vi "Main Tclk.vi"() -> ()   [LabVIEW 2018] (continued)
                          tunnel: w6883 -> [w6889 w6893]
                          tunnel: w6882 -> [w6888 w6892]
                          tunnel: [w6886 w6891] -> w6881
                          tunnel: [w6887 w6890] -> w6880
                          tunnel: w6867 -> [w6885 _]
                          tunnel: w6863 -> [w6884 _]
                          frame False {
                            n2158 = Build Array (concatenate)(w6885, w6889) -> (w6886:sgl[])
                            n2159 = Build Array (concatenate)(w6884, w6888) -> (w6887:sgl[][][])
                            n2160 = local write "FI grid array"(w6887) -> ()
                            n2161 = local write "FI array"(w6886) -> ()
                          }
                          frame True {
                            n2162 = Build Array(w6893) -> (w6891:sgl[])
                            n2163 = Build Array(w6892) -> (w6890:sgl[][][])
                            n2164 = local write "FI array"(w6891) -> ()
                            n2165 = local write "FI grid array"(w6890) -> ()
                          }
                        }
                      }
                    }
                  }
                }
                n2166 = local write "FI array tiled"(w6834) -> ()
                n2167 = local write "FI grid array tiled"(w6833) -> ()
              }
              frame #23 {
                w6915 = 1000 ("sample length")
                n2168 = local read "SEM Options"() -> (w6920:T27)
                n2169 = Unbundle By Name(w6920) -> ("Upload"=w6919:bool)
                n2170 = local read "Smart upload fail"() -> (w6943:bool)
                n2171 = local read "Milling Z voltage array"() -> (w6914:sgl[])
                n2172 = local read "Milling Z voltage (V)"() -> (w6922:sgl)
                n2173 = Compound Arithmetic op=AND(w6919, "Smart upload", w6943) -> (w6944:bool)
                n2174 = Build Array (concatenate)(w6914, w6922) -> (w6941:sgl[])
                n2175 = case shown="True" w6944 {
                  frame False {
                  }
                  frame True {
                    n2176 = local read "SEM Scan Parameters"() -> (w6949:T26)
                    n2177 = shared-variable ".\\Zeiss Library.lvlib\\Timestamp"() -> (w6950:timestamp)  [unwired: 1 in, 1 out]
                    n2178 = Unbundle By Name(w6949) -> ("Frames"=w6946:u8, "Y tiles"=w6948:u8, "X tiles"=w6947:u8)
                    n2179 = for {
                      N: w6946 -> [_]
                      tunnel: w6950 -> [w6954]
                      tunnel: w6948 -> [w6953]
                      tunnel: w6947 -> [w6952]
                      i -> [w6951]
                      n2180 = for {
                        N: w6953 -> [_]
                        tunnel: w6952 -> [w6958]
                        tunnel: w6954 -> [w6956]
                        tunnel: w6951 -> [w6955]
                        i -> [w6957]
                        n2181 = for {
                          N: w6958 -> [_]
                          tunnel: w6957 -> [w6965]
                          tunnel: w6956 -> [w6962]
                          tunnel: w6955 -> [w6961]
                          i -> [w6964]
                          w6960 = "-" ("string")
                          w6987 = "^" ("replace string (\"\")")
                          w6967 = "_" ("string")
                          n2182 = local read "Hardware Configuration"() -> (w6997:T25)
                          n2183 = local read "File Information"() -> (w6999:T31)
                          n2184 = Format Into String(w6961) -> (resulting string=w6959:string)  [unwired: 3 in, 1 out]
                          n2185 = Format Into String(w6965) -> (resulting string=w6966:string)  [unwired: 3 in, 1 out]
                          n2186 = Format Into String(w6964) -> (resulting string=w6963:string)  [unwired: 3 in, 1 out]
                          n2187 = Unbundle By Name(w6997) -> ("Machine ID"=w6996:string)
                          n2188 = Format Date/Time String(time format string (%c)="%y-%m-%d_%H%M%S", seconds (now)=w6962) -> (date/time string=w7002:string)  [unwired: 1 out]
                          n2189 = local read "SEM Options"() -> (w6982:T27)
                          n2190 = Unbundle By Name(w6999) -> ("Sample ID"=w6984:string, "File path"=w6998:path)
                          n2191 = Format Date/Time String(time format string (%c)="Y%Y\\M%m\\D%d", seconds (now)=w6962) -> (date/time string=w7007:string)  [unwired: 1 out]
                          n2192 = xnode "Match Regular Expression"("input string"=w6996, "regular expression"="/") -> ("after match"=w7006:string)  [unwired: 4 in, 4 out]
                          n2193 = Concatenate Strings(w7006, w6967, w7002, w6967, w6959, w6960, w6966, w6960, w6963, ".dat" ("string")) -> (w7008:string)
                          n2194 = Unbundle By Name(w6982) -> ("Delete after upload"=w6981:bool)
                          n2195 = Build Path(base path=w6998, name or relative path=w7007) -> (appended path=w7004:path)
                          n2196 = Build Path(base path=w7004, name or relative path=w7008) -> (appended path=w6983:path)
                          n2197 = Path To String(path=w6983) -> (string=w6990:string)
                          n2198 = shared-variable ".\\Zeiss Library.lvlib\\Upload flags path"() -> (w6969:string)  [unwired: 1 in, 1 out]
                          n2199 = Search and Replace String(replace all?=TRUE ("replace all? (F)"), input string=w6990, search string="\\", replace string=w6987) -> (result string=w6986:string)  [unwired: 4 in, 3 out]
                          n2200 = Select(t="^delete" ("replace string (\"\")"), s=w6981, f="^keep" ("replace string (\"\")")) -> (s? t:f=w6995:string)
                          n2201 = Search and Replace String(input string=w6986, search string=":", replace string=w6987) -> (result string=w6991:string)  [unwired: 5 in, 3 out]
                          n2202 = String To Path(string=w6969) -> (path=w6968:path)
                          n2203 = Concatenate Strings(w6984, "^" ("string"), w6991, w6995) -> (w6970:string)
                          n2204 = Build Path(base path=w6968, name or relative path="Filtered") -> (appended path=w6975:path)
                          n2205 = Build Path(base path=w6968, name or relative path=w6970) -> (appended path=w6980:path)
                          n2206 = File/Directory Info(path=w6975) -> (path out=w6973:path, error out=w6974:errorcluster)  [unwired: 1 in, 5 out]
                          n2207 = File/Directory Info(path=w6980) -> (path out=w6979:path, error out=w6978:errorcluster)  [unwired: 1 in, 5 out]
                          n2208 = Unbundle By Name(w6974) -> ("status"=w6972:bool)
                          n2209 = Unbundle By Name(w6978) -> ("status"=w6977:bool)
                          n2210 = case shown="True" w6972 {
                            tunnel: w6973 -> [w7009 w7011]
                            tunnel: [w7009 w7010] -> w6971
                            frame False {
                            }
                            frame True {
                              n2211 = Create Folder(path (use dialog)=w7011) -> (created path=w7010:path)  [unwired: 2 in, 2 out]
                            }
                          }
                          n2212 = case shown="False" w6977 {
                            tunnel: w6979 -> [w7015 _]
                            tunnel: w6971 -> [w7013 _]
                            tunnel: w6970 -> [w7012 _]
                            frame False {
                              n2213 = Build Path(base path=w7013, name or relative path=w7012) -> (appended path=w7014:path)
                              n2214 = Move(source path=w7015, 10:w7014) -> ()  [unwired: 3 in, 3 out]
                            }
                            frame True {
                            }
                          }
                        }
                      }
                    }
                  }
                }
                n2215 = local write "Milling Z voltage array"(w6941) -> ()
                n2216 = Array Size(array=w6941) -> (size(s)=w6916:i32)
                n2217 = Subtract(x=w6916, y=w6915) -> (x-y=w6940:i32)
                n2218 = Max & Min(x=w6916, y=w6915) -> (min(x,y)=w6917:i32)  [unwired: 1 out]
                n2219 = Array Subset(array=w6941, index=w6940, length=w6917) -> (w6942:sgl[])
                n2220 = for {
                  N: w6917 -> [_]
                  tunnel: [w6945] -> w6918 mode=indexing
                  i -> [w6945]
                }
                n2221 = call <vilib>:"Linear Fit.vi"("Y"=w6942, "X"=w6918) -> ("slope"=w6937:dbl)  [unwired: 9 in, 4 out]
                n2222 = local read "Milling para"() -> (w6935:T35)
                n2223 = local read "FIB Scan Parameters"() -> (w6938:T32)
                n2224 = Greater Or Equal?(x=w6916, y=100.0) -> (x >= y?=w6929:bool)
                n2225 = Unbundle By Name(w6935) -> ("FIB FOV (um)"=w6934:sgl)
                n2226 = Unbundle By Name(w6938) -> ("Z size (V)"=w6936:dbl)
                n2227 = Select(t=T44."Enabled" ("Disabled"), s=w6929, f=T44."Disabled and Grayed Out" ("Disabled")) -> (s? t:f=w6928:T44)
                n2228 = Divide(x=w6937, y=w6936) -> (x/y=w6933:dbl)
                n2229 = Compound Arithmetic op=MULTIPLY(w6934, sgl -1000.0 ("value"), w6933) -> (w6923:dbl)
                "Delta Z (nm)" <- w6923
                n2230 = property on="Delta Z (nm)" class="DigNum (strict)"("DisabledEnum"=w6928) -> ()  [unwired: 2 in, 2 out]
                n2231 = local read "Delta Z array"() -> (w6925:sgl[])
                n2232 = local read "SEM Specimen I array"() -> (w6927:sgl[])
                n2233 = local read "SEM Specimen I"() -> (w6894:dbl)
                n2234 = Build Array (concatenate)(w6925, w6923) -> (w6924:dbl[])
                n2235 = local write "Delta Z array"(w6924) -> ()
                n2236 = Build Array (concatenate)(w6927, w6894) -> (w6926:dbl[])
                n2237 = local write "SEM Specimen I array"(w6926) -> ()
                n2238 = local read "3D FIB-SEM Files"() -> (w6898:path)
                n2239 = local read "SEM Scan Parameters"() -> (w6903:T26)
                n2240 = Unbundle By Name(w6903) -> ("Y tiles"=w6906:u8, "X tiles"=w6904:u8)
                n2241 = Build Array(w6906, w6904) -> (w6905:u8[])
                n2242 = Quotient & Remainder(x=w6905, y=2) -> (floor(x/y)=w6901:i32[])  [unwired: 1 out]
                n2243 = Index Array(array=w6901) -> (element #1=w6912:i32, element #2=w6913:i32)  [unwired: 2 in]
                n2244 = Format Into String(w6912) -> (resulting string=w6911:string)  [unwired: 3 in, 1 out]
                n2245 = Format Into String(w6913) -> (resulting string=w6909:string)  [unwired: 3 in, 1 out]
                n2246 = Concatenate Strings("Low res_" ("string"), w6911, "-" ("string"), w6909, ".png" ("string")) -> (w6900:string)
                n2247 = Build Path(base path=w6898, name or relative path=w6900) -> (appended path=w6897:path)
                n2248 = Build Path(base path=w6898, name or relative path="Low res.png" ("string")) -> (appended path=w6896:path)
                n2249 = Copy(9:TRUE ("overwrite (F)"), 10:w6896, 11:w6897) -> ()  [unwired: 2 in, 3 out]
              }
              frame #24 {
                n2250 = local read "SEM Scan Parameters"() -> (w7139:T26)
                n2251 = local read "Auto re-engage"() -> (w7140:bool)
                n2252 = local read "Reheat from last"() -> (w7136:bool)
                n2253 = Unbundle By Name(w7139) -> ("Pixel size (nm)"=w7138:sgl, "Y tiles"=w7132:u8, "X tiles"=w7131:u8)
                n2254 = expression code="x/1000"(w7138) -> (w7137:sgl)
                n2255 = Build Array(w7132, w7131) -> (w7134:u8[])
                n2256 = Quotient & Remainder(x=w7134, y=2) -> (floor(x/y)=w7127:i32[])  [unwired: 1 out]
                n2257 = Index Array(array=w7127) -> (element #1=w7130:i32, element #2=w7129:i32)  [unwired: 2 in]
                n2258 = local read "Low res scale tiled"() -> (w7135:dbl[][])
                n2259 = Index Array(array=w7135, index (row)=w7130, index (col)=w7129) -> (element=w7128:dbl)
                n2260 = case shown="False" w7140 {
                  tunnel: w7137 -> [_ w7185]
                  tunnel: w7128 -> [_ w7184]
                  frame False {
                    n2261 = local read "Re-engage counts"() -> (w7160:u8)
                    n2262 = local read "Last re-engage count"() -> (w7162:u8)
                    n2263 = Less?(x=w7160, y=w7162) -> (x < y?=w7161:bool)
                    n2264 = case shown="True" w7161 {
                      tunnel: w7160 -> [_ w7171]
                      tunnel: w7160 -> [_ w7172]
                      frame False {
                      }
                      frame True {
                        n2265 = local read "Delta X"() -> (w7164:dbl)
                        n2266 = local read "Re-engage X shift array"() -> (w7173:dbl[])
                        n2267 = local read "SEM Scan Parameters"() -> (w7178:T26)
                        n2268 = local read "Delta Y"() -> (w7167:dbl)
                        n2269 = local read "Re-engage Y shift array"() -> (w7174:dbl[])
                        n2270 = Decrement(x=w7172) -> (x-1=w7166:u8)
                        n2271 = Decrement(x=w7171) -> (x-1=w7169:u8)
                        n2272 = Unbundle By Name(w7178) -> ("Pixel size (nm)"=w7179:sgl)
                        n2273 = Index Array(array=w7173, index=w7166) -> (element=w7165:dbl)
                        n2274 = Index Array(array=w7174, index=w7169) -> (element=w7170:dbl)
                        n2275 = expression code="x/1000"(w7179) -> (w7176:sgl)
                        n2276 = Divide(x=w7165, y=w7176) -> (x/y=w7163:dbl)
                        n2277 = Divide(x=w7170, y=w7176) -> (x/y=w7168:dbl)
                        n2278 = Subtract(x=w7164, y=w7163) -> (x-y=w7177:dbl)
                        n2279 = Subtract(x=w7167, y=w7168) -> (x-y=w7175:dbl)
                        n2280 = local read "Re-engage Delta X array"() -> (w7183:dbl[])
                        n2281 = local read "Re-engage Delta Y array"() -> (w7180:dbl[])
                        n2282 = Build Array (concatenate)(w7183, w7177) -> (w7182:dbl[])
                        n2283 = Build Array (concatenate)(w7180, w7175) -> (w7181:dbl[])
                        n2284 = local write "Re-engage Delta X array"(w7182) -> ()
                        n2285 = local write "Re-engage Delta Y array"(w7181) -> ()
                      }
                    }
                  }
                  frame True {
                    n2286 = local read "Re-engage Files"() -> (w7186:path)
                    n2287 = stacked-sequence {
                      tunnel: w7186 -> [w7187 w7214]
                      tunnel: w7185 -> [_ w7199]
                      tunnel: w7184 -> [_ w7198]
                      frame #0 {
                        n2288 = Build Path(base path=w7187, name or relative path="post.png " ("command line")) -> (appended path=w7192:path)
                        n2289 = local read "3D FIB-SEM Files"() -> (w7190:path)
                        n2290 = Build Path(base path=w7190, name or relative path="Low res.png " ("command line")) -> (appended path=w7191:path)
                        n2291 = Copy(9:TRUE ("run minimized? (F)"), 10:w7192, 11:w7191) -> ()  [unwired: 2 in, 3 out]
                      }
                      frame #1 {
                        n2292 = local read "SEM Options"() -> (w7220:T27)
                        n2293 = Unbundle By Name(w7220) -> ("Inverse PNG"=w7219:bool)
                        n2294 = call "SIFT align.vi"("Inverse PNG"=w7219, "Affine"=TRUE, "working directory"=w7214) -> ("failed"=→"Image shift search failed":bool, "Delta Y"=w7218:dbl, "Delta X"=w7215:dbl)  [unwired: 5 in, 1 out]
                        n2295 = local read "Re-engage X shift (um)"() -> (w7213:dbl)
                        n2296 = local read "Re-engage Y shift (um)"() -> (w7216:dbl)
                        n2297 = Multiply(x=w7198, y=w7215) -> (x*y=w7210:dbl)
                        n2298 = Multiply(x=w7198, y=w7218) -> (x*y=w7200:dbl)
                        n2299 = local read "Re-engage counts"() -> (w7194:u8)
                        n2300 = Add(x=w7210, y=w7213) -> (x+y=w7211:dbl)
                        "Re-engage X shift (um)" <- w7211
                        n2301 = Add(x=w7200, y=w7216) -> (x+y=w7204:dbl)
                        "Re-engage Y shift (um)" <- w7204
                        n2302 = Greater Or Equal?(x=w7194, y=u8 2) -> (x >= y?=w7197:bool)
                        n2303 = Select(t=w7210, s=w7197, f=w7211) -> (s? t:f=w7207:dbl)
                        n2304 = Select(t=w7200, s=w7197, f=w7204) -> (s? t:f=w7205:dbl)
                        n2305 = local read "Re-engage Delta X array"() -> (w7209:dbl[])
                        n2306 = local read "Re-engage Delta Y array"() -> (w7202:dbl[])
                        n2307 = Divide(x=w7207, y=w7199) -> (x/y=w7206:dbl)
                        n2308 = Divide(x=w7205, y=w7199) -> (x/y=w7201:dbl)
                        n2309 = Greater?(x=w7194, y=u8 3) -> (0:w7195:bool)
                        n2310 = Build Array (concatenate)(w7209, w7206) -> (w7208:dbl[])
                        n2311 = Build Array (concatenate)(w7202, w7201) -> (w7203:dbl[])
                        n2312 = local write "SW error warning armed"(w7195) -> ()
                        n2313 = local write "Re-engage Delta X array"(w7208) -> ()
                        n2314 = local write "Re-engage Delta Y array"(w7203) -> ()
                      }
                    }
                  }
                }
                n2315 = case shown="True" w7136 {
                  tunnel: w7128 -> [_ w7141]
                  frame False {
                  }
                  frame True {
                    n2316 = local read "Re-engage Files"() -> (w7142:path)
                    n2317 = stacked-sequence {
                      tunnel: w7142 -> [w7149 w7156]
                      tunnel: w7141 -> [_ w7152]
                      frame #0 {
                        n2318 = Build Path(base path=w7149, name or relative path="post.png " ("command line")) -> (appended path=w7144:path)
                        n2319 = local read "3D FIB-SEM Files"() -> (w7146:path)
                        n2320 = Build Path(base path=w7146, name or relative path="Low res.png " ("command line")) -> (appended path=w7145:path)
                        n2321 = Copy(9:TRUE ("run minimized? (F)"), 10:w7144, 11:w7145) -> ()  [unwired: 2 in, 3 out]
                      }
                      frame #1 {
                        n2322 = local read "SEM Options"() -> (w7158:T27)
                        n2323 = Unbundle By Name(w7158) -> ("Inverse PNG"=w7159:bool)
                        n2324 = call "SIFT align.vi"("Inverse PNG"=w7159, "Affine"=TRUE, "working directory"=w7156) -> ("failed"=w7155:bool, "Delta Y"=w7153:dbl, "Delta X"=w7154:dbl)  [unwired: 5 in, 1 out]
                        n2325 = local write "Image shift search failed"(w7155) -> ()
                        n2326 = Multiply(x=w7152, y=w7154) -> (x*y=→"X shift from last":dbl)
                        n2327 = Multiply(x=w7152, y=w7153) -> (x*y=→"Y shift from last":dbl)
                      }
                    }
                  }
                }
              }
              frame #25 {
                w7237 = u8 2 ("y")
                n2328 = local read "Re-engage Delta X array"() -> (w7240:dbl[])
                n2329 = local read "Re-engage counts"() -> (w7238:u8)
                n2330 = local read "Re-engage Delta Y array"() -> (w7235:dbl[])
                n2331 = local read "FIB"() -> (w7244:bool)
                n2332 = local read "Delta X"() -> (w7243:dbl)
                n2333 = local read "Delta Y"() -> (w7242:dbl)
                n2334 = Subtract(x=w7238, y=w7237) -> (x-y=w7234:u8)
                n2335 = local read "Delta image"() -> (w7255:dbl)
                n2336 = Index Array(array=w7240, index=w7234) -> (element=w7239:dbl)
                n2337 = Index Array(array=w7235, index=w7234) -> (element=w7236:dbl)
                n2338 = Greater Or Equal?(x=w7238, y=w7237) -> (x >= y?=w7241:bool)
                n2339 = Select(t=w7239, s=w7241, f=w7243) -> (s? t:f=w7225:dbl)
                n2340 = Select(t=w7236, s=w7241, f=w7242) -> (s? t:f=w7222:dbl)
                n2341 = case shown="True" w7244 {
                  tunnel: w7255 -> [_ w7326]
                  tunnel: w7225 -> [_ w7320]
                  tunnel: w7222 -> [_ w7319]
                  frame False {
                  }
                  frame True {
                    w7290 = enum16{"start", "end", "current"}."start" ("from (0:start)")
                    w7291 = enum16{"start", "end", "current"}."end" ("from (0:start)")
                    w7267 = 10000 ("count")
                    w7293 = -1 ("x")
                    w7350 = "," ("delimiter (Tab)")
                    w7348 = ".csv" ("string")
                    w7346 = T49."open" ("operation (0:open)")
                    w7347 = enum16{"start", "end", "current"}."end" ("from (0:start)")
                    n2342 = local read "File Information"() -> (w7349:T31)
                    n2343 = shared-variable ".\\Zeiss Library.lvlib\\Timestamp"() -> (w7328:timestamp)  [unwired: 1 in, 1 out]
                    n2344 = Unbundle By Name(w7349) -> ("File path"=w7329:path)
                    n2345 = Format Date/Time String(time format string (%c)="Y%Y\\%Y", seconds (now)=w7328) -> (date/time string=w7339:string)  [unwired: 1 out]
                    n2346 = Format Date/Time String(time format string (%c)="Y%Y\\M%m\\%Y-%m", seconds (now)=w7328) -> (date/time string=w7334:string)  [unwired: 1 out]
                    n2347 = Format Date/Time String(time format string (%c)="Y%Y\\M%m\\D%d\\%Y-%m-%d", seconds (now)=w7328) -> (date/time string=w7335:string)  [unwired: 1 out]
                    n2348 = Concatenate Strings(w7339, w7348) -> (w7333:string)
                    n2349 = Concatenate Strings(w7334, w7348) -> (w7332:string)
                    n2350 = Concatenate Strings(w7335, w7348) -> (w7331:string)
                    n2351 = Build Path(base path=w7329, name or relative path=w7333) -> (appended path=w7345:path)
                    n2352 = Build Path(base path=w7329, name or relative path=w7332) -> (appended path=w7337:path)
                    n2353 = Build Path(base path=w7329, name or relative path=w7331) -> (appended path=w7330:path)
                    n2354 = Open/Create/Replace File(file path (use dialog)=w7345, operation (0:open)=w7346) -> (refnum out=w7318:refnum<file>, error out=w7317:errorcluster)  [unwired: 1 in, 4 out]
                    n2355 = Open/Create/Replace File(file path (use dialog)=w7337, operation (0:open)=w7346) -> (refnum out=w7302:refnum<file>, error out=w7301:errorcluster)  [unwired: 1 in, 4 out]
                    n2356 = local read "SEM Scan Parameters"() -> (w7265:T26)
                    n2357 = Open/Create/Replace File(file path (use dialog)=w7330, operation (0:open)=w7346) -> (refnum out=w7310:refnum<file>, error out=w7309:errorcluster)  [unwired: 1 in, 4 out]
                    n2358 = Unbundle By Name(w7265) -> ("X tiles"=w7264:u8, "Y tiles"=w7263:u8, "Frames"=w7259:u8)
                    n2359 = Compound Arithmetic op=MULTIPLY(w7264, w7263, w7259) -> (w7261:u8)
                    n2360 = expression code="2*x-1"(w7261) -> (w7262:u8)
                    n2361 = for {
                      N: 10000 -> [_]
                      tunnel: w7317 -> [w7416]
                      tunnel: w7318 -> [w7415]
                      tunnel: [w7412] -> w7316
                      tunnel: [w7411] -> w7315
                      tunnel: [w7409] -> w7313
                      tunnel: w7291 -> [w7404]
                      shift-right: [w7401] -> _
                      shift-left: u8 0 ("count") -> [w7402]
                      tunnel: w7262 -> [w7400]
                      i -> [w7407]
                      stop <- w7399 stop-if-true
                      n2362 = expression code="-x-2"(w7407) -> (w7409:i32)
                      n2363 = Set File Position(offset (in bytes) (0)=w7409, refnum=w7415, from (0:start)=w7404, error in=w7416) -> (refnum out=w7414:refnum<file>, error out=w7413:errorcluster)
                      n2364 = Read from Text File(file (use dialog)=w7414, count=w7407, error in=w7413) -> (refnum out=w7412:refnum<file>, text=w7410:string, error out=w7411:errorcluster)  [unwired: 1 in, 1 out]
                      n2365 = Match Pattern(string=w7410, regular expression="\n") -> (offset past match=w7406:i32)  [unwired: 1 in, 3 out]
                      n2366 = Equal?(x=w7406, y=1 ("x")) -> (x = y?=w7403:bool)
                      n2367 = case shown="True" w7403 {
                        tunnel: w7402 -> [w7417 w7419]
                        tunnel: [w7417 w7418] -> w7401
                        frame False {
                        }
                        frame True {
                          n2368 = Increment(x=w7419) -> (x+1=w7418:u8)
                        }
                      }
                      n2369 = Equal?(x=w7401, y=w7400) -> (x = y?=w7399:bool)
                    }
                    n2370 = expression code="x+2"(w7261) -> (w7260:u8)
                    n2371 = Build Array(w7320, w7319, w7326) -> (w7352:dbl[])
                    n2372 = expression code="x-2"(w7313) -> (w7312:i32)
                    n2373 = Set File Position(offset (in bytes) (0)=w7313, refnum=w7316, from (0:start)=w7291, error in=w7315) -> (refnum out=w7324:refnum<file>, error out=w7325:errorcluster)
                    n2374 = Read from Text File(file (use dialog)=w7324, error in=w7325) -> (refnum out=w7289:refnum<file>, text=w7323:string, error out=w7288:errorcluster)  [unwired: 2 in, 1 out]
                    n2375 = Array To Spreadsheet String(delimiter (Tab)=w7350, array=w7352, 3:"%#g" ("format string")) -> (spreadsheet string=w7351:string)
                    n2376 = Set File Position(refnum=w7289, from (0:start)=w7290, error in=w7288) -> (refnum out=w7285:refnum<file>, error out=w7284:errorcluster)  [unwired: 1 in]
                    n2377 = Set File Position(refnum=w7302, from (0:start)=w7290, error in=w7301) -> (refnum out=w7275:refnum<file>, error out=w7271:errorcluster)  [unwired: 1 in]
                    n2378 = Set File Position(refnum=w7310, from (0:start)=w7290, error in=w7309) -> (refnum out=w7270:refnum<file>, error out=w7277:errorcluster)  [unwired: 1 in]
                    n2379 = Match Pattern(string=w7323, regular expression="\n") -> (after substring=w7322:string)  [unwired: 1 in, 3 out]
                    n2380 = Get File Size(file=w7285, error in=w7284) -> (refnum out=w7273:refnum<file>, size (in bytes)=w7282:i64, 0:w7283:errorcluster)
                    n2381 = Get File Size(file=w7275, error in=w7271) -> (refnum out=w7274:refnum<file>, size (in bytes)=w7280:i64, 0:w7272:errorcluster)
                    n2382 = Get File Size(file=w7270, error in=w7277) -> (refnum out=w7269:refnum<file>, size (in bytes)=w7278:i64, 0:w7268:errorcluster)
                    n2383 = Concatenate Strings(w7350, w7351, w7322) -> (w7327:string)
                    n2384 = Max & Min(x=w7267, y=w7282) -> (min(x,y)=w7281:i64)  [unwired: 1 out]
                    n2385 = Max & Min(x=w7267, y=w7280) -> (min(x,y)=w7279:i64)  [unwired: 1 out]
                    n2386 = Max & Min(x=w7267, y=w7278) -> (min(x,y)=w7276:i64)  [unwired: 1 out]
                    n2387 = Read from Text File(file (use dialog)=w7273, count=w7281, error in=w7283) -> (refnum out=w7287:refnum<file>, text=w7295:string, error out=w7286:errorcluster)  [unwired: 1 in, 1 out]
                    n2388 = Read from Text File(file (use dialog)=w7274, count=w7279, error in=w7272) -> (refnum out=w7300:refnum<file>, text=w7298:string, error out=w7299:errorcluster)  [unwired: 1 in, 1 out]
                    n2389 = Read from Text File(file (use dialog)=w7269, count=w7276, error in=w7268) -> (refnum out=w7307:refnum<file>, text=w7311:string, error out=w7306:errorcluster)  [unwired: 1 in, 1 out]
                    n2390 = for {
                      N: w7260 -> [_]
                      shift-right: [w7367] -> _
                      shift-left: w7295 -> [w7366]
                      tunnel: [w7365] -> w7294
                      n2391 = Match Pattern(string=w7366, regular expression="\n") -> (after substring=w7367:string, offset past match=w7365:i32)  [unwired: 1 in, 2 out]
                    }
                    n2392 = for {
                      N: w7260 -> [_]
                      shift-right: [w7382] -> _
                      shift-left: w7298 -> [w7381]
                      tunnel: [w7380] -> w7297
                      n2393 = Match Pattern(string=w7381, regular expression="\n") -> (after substring=w7382:string, offset past match=w7380:i32)  [unwired: 1 in, 2 out]
                    }
                    n2394 = for {
                      N: w7260 -> [_]
                      shift-right: [w7397] -> _
                      shift-left: w7311 -> [w7396]
                      tunnel: [w7395] -> w7308
                      n2395 = Match Pattern(string=w7396, regular expression="\n") -> (after substring=w7397:string, offset past match=w7395:i32)  [unwired: 1 in, 2 out]
                    }
                    n2396 = Not Equal?(x=w7293, y=w7294) -> (x != y?=w7292:bool)
                    n2397 = Not Equal?(x=w7293, y=w7297) -> (x != y?=w7296:bool)
                    n2398 = Not Equal?(x=w7293, y=w7308) -> (x != y?=w7305:bool)
                    n2399 = case shown="True" w7292 {
                      tunnel: w7347 -> [_ w7364]
                      tunnel: [w7355 w7361] -> w7344
                      tunnel: [w7354 w7360] -> w7343
                      tunnel: w7327 -> [_ w7359]
                      tunnel: w7287 -> [w7355 w7358]
                      tunnel: w7286 -> [w7354 w7357]
                      tunnel: w7312 -> [_ w7356]
                      frame False {
                      }
                      frame True {
                        n2400 = Set File Position(offset (in bytes) (0)=w7356, refnum=w7358, from (0:start)=w7364, error in=w7357) -> (refnum out=w7362:refnum<file>, error out=w7363:errorcluster)
                        n2401 = Write to Text File(file (use dialog)=w7362, text=w7359, error in=w7363) -> (refnum out=w7361:refnum<file>, error out=w7360:errorcluster)  [unwired: 2 out]
                      }
                    }
                    n2402 = case shown="False" w7296 {
                      tunnel: w7347 -> [_ w7379]
                      tunnel: [w7369 w7378] -> w7342
                      tunnel: [w7370 w7377] -> w7341
                      tunnel: w7327 -> [_ w7374]
                      tunnel: w7312 -> [_ w7373]
                      tunnel: w7300 -> [w7370 w7372]
                      tunnel: w7299 -> [w7369 w7371]
                      frame False {
                      }
                      frame True {
                        n2403 = Set File Position(offset (in bytes) (0)=w7373, refnum=w7372, from (0:start)=w7379, error in=w7371) -> (refnum out=w7376:refnum<file>, error out=w7375:errorcluster)
                        n2404 = Write to Text File(file (use dialog)=w7376, text=w7374, error in=w7375) -> (refnum out=w7377:refnum<file>, error out=w7378:errorcluster)  [unwired: 2 out]
                      }
                    }
                    n2405 = case shown="True" w7305 {
                      tunnel: w7347 -> [_ w7394]
                      tunnel: w7327 -> [_ w7392]
                      tunnel: w7312 -> [_ w7391]
                      tunnel: w7307 -> [w7385 w7389]
                      tunnel: w7306 -> [w7384 w7388]
                      tunnel: [w7385 w7387] -> w7304
                      tunnel: [w7384 w7386] -> w7303
                      frame False {
                      }
                      frame True {
                        n2406 = Set File Position(offset (in bytes) (0)=w7391, refnum=w7389, from (0:start)=w7394, error in=w7388) -> (refnum out=w7393:refnum<file>, error out=w7390:errorcluster)
                        n2407 = Write to Text File(file (use dialog)=w7393, text=w7392, error in=w7390) -> (refnum out=w7387:refnum<file>, error out=w7386:errorcluster)  [unwired: 2 out]
                      }
                    }
                    n2408 = Close File(refnum=w7344, error in=w7343) -> ()  [unwired: 2 out]
                    n2409 = Close File(refnum=w7341, error in=w7342) -> ()  [unwired: 2 out]
                    n2410 = Close File(refnum=w7304, error in=w7303) -> ()  [unwired: 2 out]
                  }
                }
                n2411 = To Single Precision Float(number=w7255) -> (single precision float=w7232:sgl)
                n2412 = local read "Delta X array"() -> (w7258:sgl[])
                n2413 = local read "Delta X sum array"() -> (w7253:sgl[])
                n2414 = local read "Delta Y array"() -> (w7256:sgl[])
                n2415 = local read "Delta Y sum array"() -> (w7246:sgl[])
                n2416 = local read "Delta image array"() -> (w7257:sgl[])
                n2417 = Build Array (concatenate)(w7258, w7225) -> (w7231:dbl[])
                n2418 = Build Array (concatenate)(w7256, w7222) -> (w7229:dbl[])
                n2419 = Array Size(array=w7253) -> (size(s)=w7254:i32)
                n2420 = Array Size(array=w7246) -> (size(s)=w7247:i32)
                n2421 = Build Array (concatenate)(w7257, w7232) -> (w7233:sgl[])
                n2422 = local write "Delta X array"(w7231) -> ()
                n2423 = local write "Delta Y array"(w7229) -> ()
                n2424 = Decrement(x=w7254) -> (x-1=w7252:i32)
                n2425 = Decrement(x=w7247) -> (x-1=w7248:i32)
                n2426 = local write "Delta image array"(w7233) -> ()
                n2427 = Index Array(array=w7253, index=w7252) -> (element=w7251:sgl)
                n2428 = Index Array(array=w7246, index=w7248) -> (element=w7249:sgl)
                n2429 = Add(x=w7251, y=w7225) -> (x+y=w7250:dbl)
                n2430 = Add(x=w7249, y=w7222) -> (x+y=w7245:dbl)
                n2431 = local read "Delta X array for stop limit"() -> (w7226:sgl[])
                n2432 = local read "Delta Y array for stop limit"() -> (w7223:sgl[])
                n2433 = Build Array (concatenate)(w7253, w7250) -> (w7230:dbl[])
                n2434 = Build Array (concatenate)(w7246, w7245) -> (w7228:dbl[])
                n2435 = local write "Delta X sum array"(w7230) -> ()
                n2436 = local write "Delta Y sum array"(w7228) -> ()
                n2437 = Build Array (concatenate)(w7226, w7225) -> (w7227:dbl[])
                n2438 = Build Array (concatenate)(w7223, w7222) -> (w7224:dbl[])
                n2439 = local write "Delta X array for stop limit"(w7227) -> ()
                n2440 = local write "Delta Y array for stop limit"(w7224) -> ()
              }
              frame #26 {
                n2441 = local read "Faraday Cup before mill"() -> (w7454:sgl)
                n2442 = local read "Faraday Cup array"() -> (w7451:sgl[])
                n2443 = local read "Milling para"() -> (w7449:T35)
                n2444 = Unbundle By Name(w7449) -> ("FIB PID on"=w7448:bool, "FIB PID measured"=w7447:u8)
                n2445 = Array Size(array=w7451) -> (size(s)=w7453:i32)
                n2446 = Greater Or Equal?(x=w7453, y=10 ("x")) -> (x >= y?=w7450:bool)
                n2447 = case shown="True" w7450 {
                  tunnel: w7454 -> [w7703 w7707]
                  tunnel: w7451 -> [_ w7718]
                  tunnel: [w7696 w7716] -> _
                  tunnel: [w7696 w7705] -> w7446
                  frame False {
                    w7704 = sgl 0.5 ("y")
                    w7696 = FALSE
                    n2448 = local read "Faraday Cup low limit array"() -> (w7701:sgl[])
                    n2449 = local read "Faraday Cup high limit array"() -> (w7699:sgl[])
                    n2450 = Subtract(x=w7703, y=w7704) -> (x-y=w7700:sgl)
                    n2451 = Add(x=w7704, y=w7703) -> (x+y=w7697:sgl)
                    n2452 = Build Array (concatenate)(w7701, w7700) -> (w7702:sgl[])
                    n2453 = Build Array (concatenate)(w7699, w7697) -> (w7698:sgl[])
                    n2454 = local write "Faraday Cup low limit array"(w7702) -> ()
                    n2455 = local write "Faraday Cup high limit array"(w7698) -> ()
                  }
                  frame True {
                    n2456 = call "Auto limits.vi"("Minimum half range"=0.5, "# of interquartile range or stdev"=6.0 ("# of sigma"), "Length"=1000, "Input array"=w7718) -> ("Low limit"=w7706:dbl, "High limit"=w7713:dbl)  [unwired: 5 in, 1 out]
                    n2457 = Less Or Equal?(x=w7707, y=w7706) -> (x <= y?=w7705:bool)
                    n2458 = local read "Faraday Cup high limit array"() -> (w7714:sgl[])
                    n2459 = local read "Faraday Cup low limit array"() -> (w7710:sgl[])
                    n2460 = To Single Precision Float(number=w7713) -> (single precision float=w7708:sgl)
                    n2461 = To Single Precision Float(number=w7706) -> (single precision float=w7709:sgl)
                    n2462 = In Range and Coerce(upper limit=w7708, x=w7707, lower limit=w7709) -> (In Range?=w7717:bool)  [unwired: 1 out]
                    n2463 = Build Array (concatenate)(w7714, w7708) -> (w7712:sgl[])
                    n2464 = Build Array (concatenate)(w7710, w7709) -> (w7711:sgl[])
                    n2465 = Not(x=w7717) -> (.not. x?=w7716:bool)
                    n2466 = local write "Faraday Cup high limit array"(w7712) -> ()
                    n2467 = local write "Faraday Cup low limit array"(w7711) -> ()
                  }
                }
                "Faraday cup I low" <- w7446
                n2468 = case shown="True" w7448 {
                  tunnel: w7447 -> [_ w7503]
                  frame False {
                    n2469 = local read "Specimen I array"() -> (w7499:sgl[])
                    n2470 = local read "Beam Dump 1 array"() -> (w7482:sgl[])
                    n2471 = local read "Beam Dump 2 array"() -> (w7475:sgl[])
                    n2472 = local read "Milling I array"() -> (w7458:sgl[])
                    n2473 = call "Auto limits.vi"("Minimum half range"=0.5, "# of interquartile range or stdev"=6.0 ("# of sigma"), "Length"=100, "Input array"=w7499) -> ("Low limit"=w7497:dbl, "High limit"=w7498:dbl)  [unwired: 5 in, 1 out]
                    n2474 = call "Auto limits.vi"("Minimum half range"=0.5, "# of interquartile range or stdev"=6.0 ("# of sigma"), "Length"=100, "Input array"=w7482) -> ("Low limit"=w7484:dbl, "High limit"=w7483:dbl)  [unwired: 5 in, 1 out]
                    n2475 = call "Auto limits.vi"("Minimum half range"=0.5, "# of interquartile range or stdev"=6.0 ("# of sigma"), "Length"=100, "Input array"=w7475) -> ("Low limit"=w7473:dbl, "High limit"=w7474:dbl)  [unwired: 5 in, 1 out]
                    n2476 = call "Auto limits.vi"("Minimum half range"=0.5, "# of interquartile range or stdev"=6.0 ("# of sigma"), "Length"=100, "Input array"=w7458) -> ("Low limit"=w7460:dbl, "High limit"=w7459:dbl)  [unwired: 5 in, 1 out]
                    n2477 = To Single Precision Float(number=w7498) -> (single precision float=w7492:sgl)
                    n2478 = To Single Precision Float(number=w7497) -> (single precision float=w7491:sgl)
                    n2479 = To Single Precision Float(number=w7483) -> (single precision float=w7489:sgl)
                    n2480 = To Single Precision Float(number=w7484) -> (single precision float=w7490:sgl)
                    n2481 = To Single Precision Float(number=w7474) -> (single precision float=w7468:sgl)
                    n2482 = To Single Precision Float(number=w7473) -> (single precision float=w7467:sgl)
                    n2483 = To Single Precision Float(number=w7459) -> (single precision float=w7465:sgl)
                    n2484 = To Single Precision Float(number=w7460) -> (single precision float=w7466:sgl)
                    n2485 = local read "Specimen I high limit array"() -> (w7494:sgl[])
                    n2486 = local read "Specimen I low limit array"() -> (w7495:sgl[])
                    n2487 = local read "BD1 high limit array"() -> (w7487:sgl[])
                    n2488 = local read "BD2 high limit array"() -> (w7470:sgl[])
                    n2489 = local read "Milling I high limit array"() -> (w7463:sgl[])
                    n2490 = local read "BD1 low limit array"() -> (w7486:sgl[])
                    n2491 = local read "BD2 low limit array"() -> (w7471:sgl[])
                    n2492 = local read "Milling I low limit array"() -> (w7462:sgl[])
                    n2493 = Build Array (concatenate)(w7494, w7492) -> (w7493:sgl[])
                    n2494 = Build Array (concatenate)(w7495, w7491) -> (w7496:sgl[])
                    n2495 = Build Array (concatenate)(w7487, w7489) -> (w7488:sgl[])
                    n2496 = Build Array (concatenate)(w7486, w7490) -> (w7485:sgl[])
                    n2497 = Build Array (concatenate)(w7470, w7468) -> (w7469:sgl[])
                    n2498 = Build Array (concatenate)(w7471, w7467) -> (w7472:sgl[])
                    n2499 = Build Array (concatenate)(w7463, w7465) -> (w7464:sgl[])
                    n2500 = Build Array (concatenate)(w7462, w7466) -> (w7461:sgl[])
                    n2501 = local write "Specimen I high limit array"(w7493) -> ()
                    n2502 = local write "Specimen I low limit array"(w7496) -> ()
                    n2503 = local write "BD1 high limit array"(w7488) -> ()
                    n2504 = local write "BD2 high limit array"(w7469) -> ()
                    n2505 = local write "Milling I high limit array"(w7464) -> ()
                    n2506 = local write "BD1 low limit array"(w7485) -> ()
                    n2507 = local write "BD2 low limit array"(w7472) -> ()
                    n2508 = local write "Milling I low limit array"(w7461) -> ()
                  }
                  frame True {
                    n2509 = case shown="100, Default" w7503 {
                      frame 0 {
                        n2510 = local read "Beam Dump 1 array"() -> (w7531:sgl[])
                        n2511 = local read "Beam Dump 2 array"() -> (w7524:sgl[])
                        n2512 = local read "Milling I array"() -> (w7507:sgl[])
                        n2513 = call "Auto limits.vi"("Minimum half range"=0.5, "# of interquartile range or stdev"=6.0 ("# of sigma"), "Length"=100, "Input array"=w7531) -> ("Low limit"=w7533:dbl, "High limit"=w7532:dbl)  [unwired: 5 in, 1 out]
                        n2514 = call "Auto limits.vi"("Minimum half range"=0.5, "# of interquartile range or stdev"=6.0 ("# of sigma"), "Length"=100, "Input array"=w7524) -> ("Low limit"=w7522:dbl, "High limit"=w7523:dbl)  [unwired: 5 in, 1 out]
                        n2515 = call "Auto limits.vi"("Minimum half range"=0.5, "# of interquartile range or stdev"=6.0 ("# of sigma"), "Length"=100, "Input array"=w7507) -> ("Low limit"=w7509:dbl, "High limit"=w7508:dbl)  [unwired: 5 in, 1 out]
                        n2516 = To Single Precision Float(number=w7532) -> (single precision float=w7538:sgl)
                        n2517 = To Single Precision Float(number=w7533) -> (single precision float=w7539:sgl)
                        n2518 = To Single Precision Float(number=w7523) -> (single precision float=w7517:sgl)
                        n2519 = To Single Precision Float(number=w7522) -> (single precision float=w7516:sgl)
                        n2520 = To Single Precision Float(number=w7508) -> (single precision float=w7514:sgl)
                        n2521 = To Single Precision Float(number=w7509) -> (single precision float=w7515:sgl)
                        n2522 = local read "BD1 high limit array"() -> (w7536:sgl[])
                        n2523 = local read "BD2 high limit array"() -> (w7519:sgl[])
                        n2524 = local read "Milling I high limit array"() -> (w7512:sgl[])
                        n2525 = local read "BD1 low limit array"() -> (w7535:sgl[])
                        n2526 = local read "BD2 low limit array"() -> (w7520:sgl[])
                        n2527 = local read "Milling I low limit array"() -> (w7511:sgl[])
                        n2528 = Build Array (concatenate)(w7536, w7538) -> (w7537:sgl[])
                        n2529 = Build Array (concatenate)(w7535, w7539) -> (w7534:sgl[])
                        n2530 = Build Array (concatenate)(w7519, w7517) -> (w7518:sgl[])
                        n2531 = Build Array (concatenate)(w7520, w7516) -> (w7521:sgl[])
                        n2532 = Build Array (concatenate)(w7512, w7514) -> (w7513:sgl[])
                        n2533 = Build Array (concatenate)(w7511, w7515) -> (w7510:sgl[])
                        n2534 = local write "BD1 high limit array"(w7537) -> ()
                        n2535 = local write "BD2 high limit array"(w7518) -> ()
                        n2536 = local write "Milling I high limit array"(w7513) -> ()
                        n2537 = local write "BD1 low limit array"(w7534) -> ()
                        n2538 = local write "BD2 low limit array"(w7521) -> ()
                        n2539 = local write "Milling I low limit array"(w7510) -> ()
                      }
                      frame 1 {
                        n2540 = local read "Specimen I array"() -> (w7572:sgl[])
                        n2541 = local read "Beam Dump 2 array"() -> (w7560:sgl[])
                        n2542 = local read "Milling I array"() -> (w7543:sgl[])
                        n2543 = call "Auto limits.vi"("Minimum half range"=0.5, "# of interquartile range or stdev"=6.0 ("# of sigma"), "Length"=100, "Input array"=w7572) -> ("Low limit"=w7570:dbl, "High limit"=w7571:dbl)  [unwired: 5 in, 1 out]
                        n2544 = call "Auto limits.vi"("Minimum half range"=0.5, "# of interquartile range or stdev"=6.0 ("# of sigma"), "Length"=100, "Input array"=w7560) -> ("Low limit"=w7558:dbl, "High limit"=w7559:dbl)  [unwired: 5 in, 1 out]
                        n2545 = call "Auto limits.vi"("Minimum half range"=0.5, "# of interquartile range or stdev"=6.0 ("# of sigma"), "Length"=100, "Input array"=w7543) -> ("Low limit"=w7545:dbl, "High limit"=w7544:dbl)  [unwired: 5 in, 1 out]
                        n2546 = To Single Precision Float(number=w7571) -> (single precision float=w7565:sgl)
                        n2547 = To Single Precision Float(number=w7570) -> (single precision float=w7564:sgl)
                        n2548 = To Single Precision Float(number=w7559) -> (single precision float=w7553:sgl)
                        n2549 = To Single Precision Float(number=w7558) -> (single precision float=w7552:sgl)
                        n2550 = To Single Precision Float(number=w7544) -> (single precision float=w7550:sgl)
                        n2551 = To Single Precision Float(number=w7545) -> (single precision float=w7551:sgl)
                        n2552 = local read "Specimen I high limit array"() -> (w7567:sgl[])
                        n2553 = local read "Specimen I low limit array"() -> (w7568:sgl[])
                        n2554 = local read "BD2 high limit array"() -> (w7555:sgl[])
                        n2555 = local read "Milling I high limit array"() -> (w7548:sgl[])
                        n2556 = local read "BD2 low limit array"() -> (w7556:sgl[])
                        n2557 = local read "Milling I low limit array"() -> (w7547:sgl[])
                        n2558 = Build Array (concatenate)(w7567, w7565) -> (w7566:sgl[])
                        n2559 = Build Array (concatenate)(w7568, w7564) -> (w7569:sgl[])
                        n2560 = Build Array (concatenate)(w7555, w7553) -> (w7554:sgl[])
                        n2561 = Build Array (concatenate)(w7556, w7552) -> (w7557:sgl[])
                        n2562 = Build Array (concatenate)(w7548, w7550) -> (w7549:sgl[])
                        n2563 = Build Array (concatenate)(w7547, w7551) -> (w7546:sgl[])
                        n2564 = local write "Specimen I high limit array"(w7566) -> ()
                        n2565 = local write "Specimen I low limit array"(w7569) -> ()
                        n2566 = local write "BD2 high limit array"(w7554) -> ()
                        n2567 = local write "Milling I high limit array"(w7549) -> ()
                        n2568 = local write "BD2 low limit array"(w7557) -> ()
                        n2569 = local write "Milling I low limit array"(w7546) -> ()
                      }
